vi "Pointer producer consumer Sound.vi"(0 "Sound":bool, 3 "Numeric":i32) -> ()   [LabVIEW 2014]
panel:
  in  "frequency (Hz)":u32=500
  in  "use system alert? (T)":bool
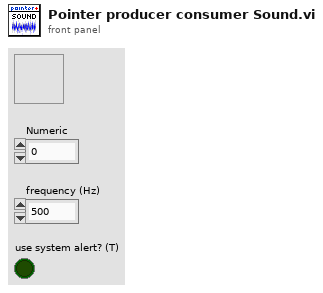
[diagram p1: front panel]
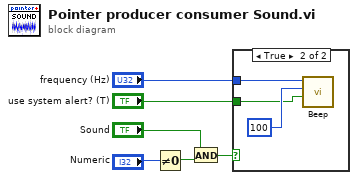
[diagram p0: block diagram]
diagram:
  n1 = Not Equal To 0?(x="Numeric") -> (x != 0?=w6:bool)
  n2 = And(x="Sound", y=w6) -> (x .and. y?=w3:bool)
  n3 = case shown="True" w3 {
    tunnel: "frequency (Hz)" -> [_ w8]
    tunnel: "use system alert? (T)" -> [_ w7]
    frame False {
    }
    frame True {
      n4 = call <vilib>:"Beep.vi"("use system alert? (T)"=w7, "duration (msec)"=u32 100, "frequency (Hz)"=w8) -> ()  [unwired: 9 in]
    }
  }
